vi "Enqueue - ClusterQueue.vi"   [LabVIEW 2010]
doc: "This VI handles all enqueue functions available:\n\nEnqueue - ClusterCommand (enqueues command only, no data)\nEnqueue - ClusterBoth (enqueues command and data)\nEnqueue - Multiple Clusters (enqueues an array of command & data clusters)\nEnqueue - Multiple Commmands (enqueues an array of commands, no data)"
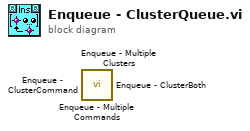
[diagram p0: block diagram]
diagram:
  n1 = call <userlib>:"Enqueue - Multiple Commands.vi"() -> ()  [unwired: 10 in, 2 out]
  n2 = call <userlib>:"Enqueue - Multiple Clusters.vi"() -> ()  [unwired: 10 in, 2 out]
  n3 = call <userlib>:"Enqueue - ClusterCommand.vi"() -> ()  [unwired: 10 in, 2 out]
  n4 = call <userlib>:"Enqueue - ClusterBoth.vi"() -> ()  [unwired: 10 in, 2 out]
